vi "UNIT8Array to BoolArray.vi"(1 "Input Array (UINT_8)":u8[](array[numeric])) -> (0 "Output Array (Bool)":bool[](array[boolean]))   [LabVIEW 2014]
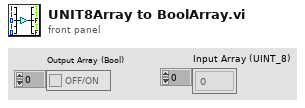
[diagram p1: front panel]
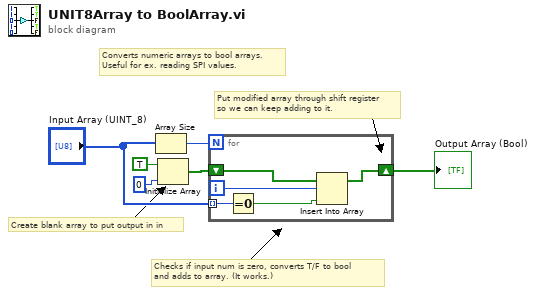
[diagram p0: block diagram]
diagram:
  # "Put modified array through shift register\nso we can keep adding to it."
  # "Checks if input num is zero, converts T/F to bool\nand adds to array. (It works.)"
  # "Create blank array to put output in in"
  # "Converts numeric arrays to bool arrays.\nUseful for ex. reading SPI values."
  n1 = Array Size(array="Input Array (UINT_8)") -> (size(s)=w6:i32)
  n2 = Initialize Array(TRUE, 0) -> (w5:bool[])
  n3 = for {
    N: w6 -> [_]
    tunnel: "Input Array (UINT_8)" -> [w8] mode=indexing
    shift-right: [w9] -> w1
    shift-left: w5 -> [w10]
    i -> [w11]
    n4 = Equal To 0?(x=w8) -> (x = 0?=w7:bool)
    n5 = Insert Into Array(array=w10, index=w11, new element=w7) -> (w9:bool[])
  }
  "Output Array (Bool)" <- w1
